vi "Set Numeric.vi"(8 "error in (no error)":errorcluster, 10 "Boolean":bool, 11 "Element A in":refnum<class "Element A.lvclass">) -> (0 "error out":errorcluster, 3 "Element A out":refnum<class "Element A.lvclass">)   [LabVIEW 2020, in "Array Example.lvlib" / "Element A.lvclass"]
uses:
  Element A.lvclass
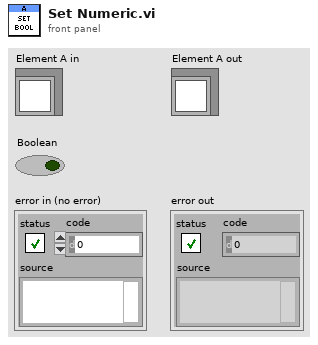
[diagram p1: front panel]
types:
  T1 = typedef "Array Example.lvlib/Element A.lvclass/Ref.ctl" = cluster{"Boolean":bool}
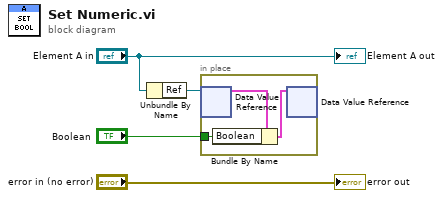
[diagram p0: block diagram]
diagram:
  n1 = Unbundle By Name("Element A in") -> ("Ref"=w3:refnum<data-value>)
  n2 = in-place {
    in-place-border: "Boolean" -> [w5]
    n3 = in-place-dvr #1(w3) -> (w7:T1)  [unwired: 1 out]
    n4 = Bundle By Name(cluster=w7, "Boolean"=w5) -> (w6:T1)
    n5 = in-place-dvr #1(w6) -> ()  [unwired: 2 out]
  }
  "error out" <- "error in (no error)"
  "Element A out" <- "Element A in"
